vi "Run Step.vi"(0 "Profile":string[][](array[string]), 1 "Current Step in":i32, 2 "# of Steps":i32, 3 "Cycles Completed in":u32, 4 "Pumps Present":T1) -> (12 "Bank1State":u16, 14 "Bank2State":u16, 16 "LS Freq":dbl, 18 "LS Duty":dbl, 20 "PS Cmd":dbl, 21 "Press Cmd":dbl, 22 "Ignition Relays":T1, 23 "Current Step out":i32, 24 "Cycles Completed out":u32, 25 "Step Time":dbl, 26 "Controller CMDs":dbl[](array[numeric]), 27 "Power Relays":T1)   [LabVIEW 2013]
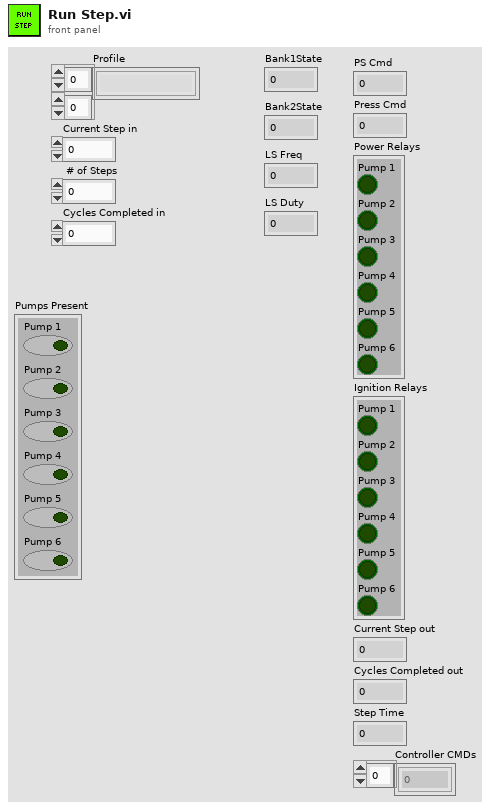
[diagram p1: front panel]
types:
  T1 = cluster{"Pump 1":bool, "Pump 2":bool, "Pump 3":bool, "Pump 4":bool, "Pump 5":bool, "Pump 6":bool}
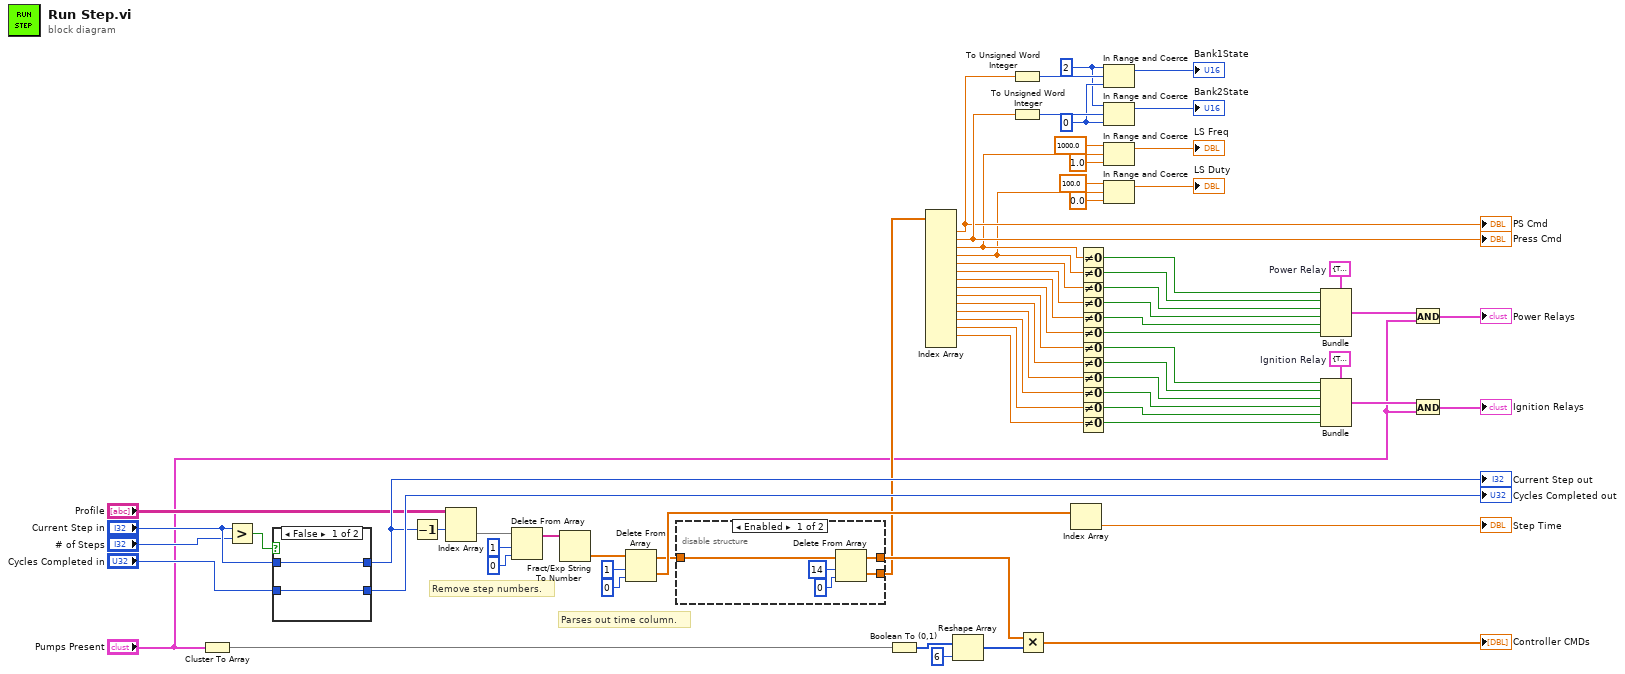
[diagram p0: block diagram]
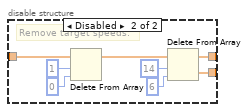
[diagram p2: hidden frame]
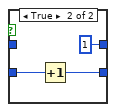
[diagram p3: hidden frame]
diagram:
  w7 = u16 2
  w8 = u16 0
  w39 = T1 {"Pump 1"=TRUE, "Pump 2"=TRUE, "Pump 3"=TRUE, "Pump 4"=TRUE, "Pump 5"=TRUE, "Pump 6"=TRUE}  # Ignition Relay
  w40 = T1 {"Pump 1"=TRUE, "Pump 2"=TRUE, "Pump 3"=TRUE, "Pump 4"=TRUE, "Pump 5"=TRUE, "Pump 6"=TRUE}  # Power Relay
  # "Parses out time column."
  # "Remove step numbers."
  n1 = Cluster To Array(cluster="Pumps Present") -> (array=w23:bool[])
  n2 = Greater?(x="Current Step in", y="# of Steps") -> (0:w66:bool)
  n3 = case shown="False" w66 {
    tunnel: [w72 1 ("Current Step")] -> w68
    tunnel: "Current Step in" -> [w72 _]
    tunnel: "Cycles Completed in" -> [w71 w74]
    tunnel: [w71 w73] -> w70
    frame False {
    }
    frame True {
      n4 = Increment(x=w74) -> (x+1=w73:u32)
    }
  }
  "Cycles Completed out" <- w70
  "Current Step out" <- w68
  n5 = Decrement(x=w68) -> (x-1=w55:i32)
  n6 = Index Array(array="Profile", index (row)=w55) -> (element=w56:string[])  [unwired: 1 in]
  n7 = Delete From Array(array=w56, length=1, index=0 ("length")) -> (array with subset deleted=w59:string[])  [unwired: 1 out]
  n8 = Fract/Exp String To Number(string=w59) -> (number=w62:dbl[])  [unwired: 3 in, 1 out]
  n9 = Delete From Array(array=w62, length=1, index=0 ("length")) -> (deleted portion=w63:dbl[], array with subset deleted=w22:dbl[])
  n10 = disable-structure shown="Enabled" {
    disable-tunnel: [w78 w86] -> w53
    disable-tunnel: [w77 w85] -> w51
    disable-tunnel: w22 -> [w76 w82]
    frame Enabled {
      n11 = Delete From Array(array=w76, length=14, index=0) -> (deleted portion=w77:dbl[], array with subset deleted=w78:dbl[])
    }
    frame Disabled {
      # "Remove target speeds."
      n12 = Delete From Array(array=w82, length=1, index=0 ("length")) -> (array with subset deleted=w81:dbl[])  [unwired: 1 out]
      n13 = Delete From Array(array=w81, length=14, index=6) -> (deleted portion=w85:dbl[], array with subset deleted=w86:dbl[])
    }
  }
  n14 = Boolean To (0,1)(Boolean=w23) -> (0, 1=w26:i16[])
  n15 = Index Array(array=w51) -> (element #1=w11:dbl, element #2=w12:dbl, element #3=w2:dbl, element #4=w1:dbl, element #5=w49:dbl, element #6=w50:dbl, element #7=w48:dbl, element #8=w47:dbl, element #9=w46:dbl, element #10=w44:dbl, element #11=w45:dbl, element #12=w43:dbl, element #13=w42:dbl, element #14=w41:dbl)  [unwired: 15 in, 1 out]
  "PS Cmd" <- w11
  "Press Cmd" <- w12
  n16 = Reshape Array(w26, 6 ("dimension size")) -> (w25:i16[])
  n17 = To Unsigned Word Integer(number=w11) -> (unsigned 16bit integer=w10:u16)
  n18 = To Unsigned Word Integer(number=w12) -> (unsigned 16bit integer=w9:u16)
  n19 = Multiply(x=w53, y=w25) -> (x*y=→"Controller CMDs":dbl[])
  n20 = Index Array(array=w63) -> (element=→"Step Time":dbl)  [unwired: 1 in]
  n21 = Not Equal To 0?(x=w2) -> (x != 0?=w38:bool)
  n22 = Not Equal To 0?(x=w1) -> (x != 0?=w37:bool)
  n23 = Not Equal To 0?(x=w49) -> (x != 0?=w36:bool)
  n24 = Not Equal To 0?(x=w50) -> (x != 0?=w35:bool)
  n25 = Not Equal To 0?(x=w48) -> (x != 0?=w34:bool)
  n26 = Not Equal To 0?(x=w47) -> (x != 0?=w33:bool)
  n27 = Not Equal To 0?(x=w46) -> (x != 0?=w32:bool)
  n28 = Not Equal To 0?(x=w44) -> (x != 0?=w31:bool)
  n29 = Not Equal To 0?(x=w45) -> (x != 0?=w30:bool)
  n30 = Not Equal To 0?(x=w43) -> (x != 0?=w28:bool)
  n31 = Not Equal To 0?(x=w42) -> (x != 0?=w29:bool)
  n32 = Not Equal To 0?(x=w41) -> (x != 0?=w27:bool)
  n33 = In Range and Coerce(upper limit=w7, x=w10, lower limit=w8) -> (coerced(x)=→"Bank1State":u16)  [unwired: 1 out]
  n34 = In Range and Coerce(upper limit=w7, x=w9, lower limit=w8) -> (coerced(x)=→"Bank2State":u16)  [unwired: 1 out]
  n35 = In Range and Coerce(upper limit=1000.0, x=w2, lower limit=1.0) -> (coerced(x)=→"LS Freq":dbl)  [unwired: 1 out]
  n36 = In Range and Coerce(upper limit=100.0, x=w1, lower limit=0.0) -> (coerced(x)=→"LS Duty":dbl)  [unwired: 1 out]
  n37 = Bundle(cluster=w40, "Pump 1"=w38, "Pump 2"=w37, "Pump 3"=w36, "Pump 4"=w35, "Pump 5"=w34, "Pump 6"=w33) -> (w21:T1)
  n38 = Bundle(cluster=w39, "Pump 1"=w32, "Pump 2"=w31, "Pump 3"=w30, "Pump 4"=w28, "Pump 5"=w29, "Pump 6"=w27) -> (w19:T1)
  n39 = And(x=w21, y="Pumps Present") -> (x .and. y?=→"Power Relays":T1)
  n40 = And(x=w19, y="Pumps Present") -> (x .and. y?=→"Ignition Relays":T1)
